vi "Init.vi"(0 "Measurement3D in":refnum<class "Measurement3D.lvclass">, 1 "Instrument 1.lvclass":refnum<class "Instrument.lvclass">, 2 "Instrument 2.lvclass":refnum<class "Instrument.lvclass">, 3 "Instrument 3.lvclass":refnum<class "Instrument.lvclass">, 4 "Inner Loop":T2, 5 "Outer Loop":T1, 7 "error in (no error)":errorcluster) -> (20 "Measurement3D out":refnum<class "Measurement3D.lvclass">, 27 "error out":errorcluster)   [LabVIEW 2014, in "Measurement3D.lvclass"]
uses:
  Measurement3D.lvclass
  Instrument/Instrument/Instrument.lvclass
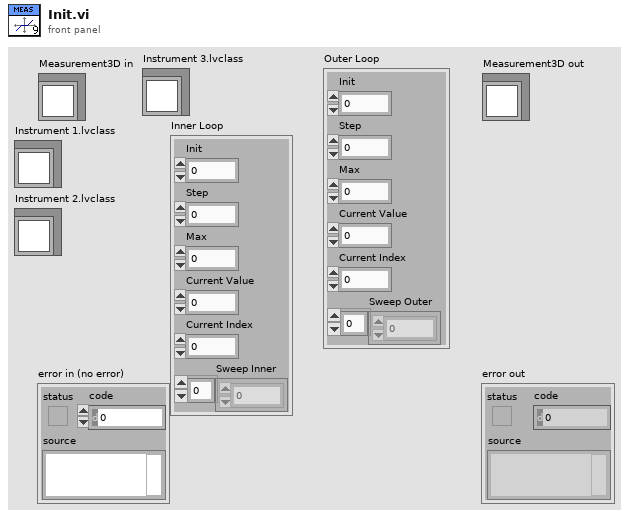
[diagram p1: front panel]
types:
  T1 = cluster{"Init":dbl, "Step":dbl, "Max":dbl, "Current Value":dbl, "Current Index":dbl, "Sweep Outer":dbl[]}
  T2 = cluster{"Init":dbl, "Step":dbl, "Max":dbl, "Current Value":dbl, "Current Index":dbl, "Sweep Inner":dbl[]}
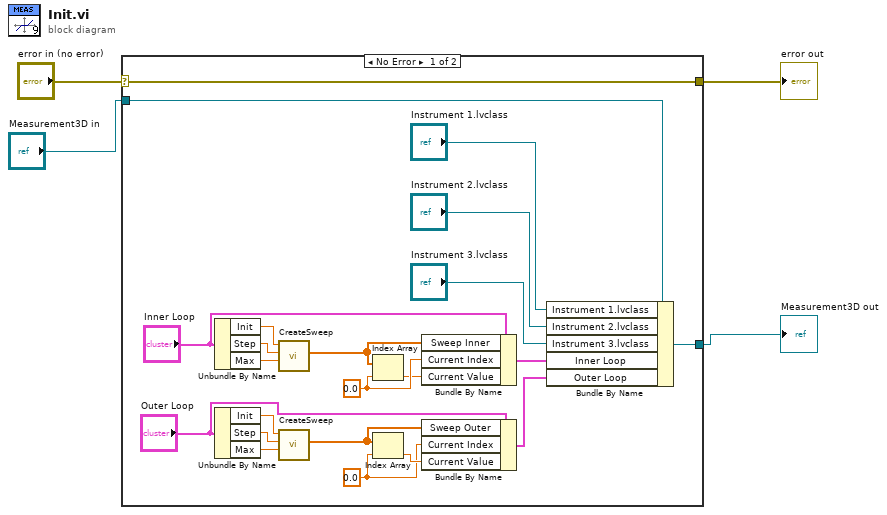
[diagram p0: block diagram]
diagram:
  n1 = case shown="No Error" "error in (no error)" {
    selector: "error in (no error)" -> [w26 w28]
    tunnel: [w26 w28] -> w3
    tunnel: [w21 w27] -> w1
    tunnel: "Measurement3D in" -> [w25 w27]
    frame No Error {
      w6 = 0.0 ("Current Index")
      w9 = 0.0 ("Current Index")
      n2 = Unbundle By Name("Inner Loop") -> ("Init"=w19:dbl, "Step"=w18:dbl, "Max"=w17:dbl)
      n3 = Unbundle By Name("Outer Loop") -> ("Init"=w15:dbl, "Step"=w14:dbl, "Max"=w13:dbl)
      n4 = call "CreateSweep.vi"("Max"=w17, "Step"=w18, "Init Value"=w19) -> ("Array"=w10:dbl[])  [unwired: 8 in]
      n5 = call "CreateSweep.vi"("Max"=w13, "Step"=w14, "Init Value"=w15) -> ("Array"=w5:dbl[])  [unwired: 8 in]
      n6 = Index Array(array=w10, index=w9) -> (element=w8:dbl)
      n7 = Index Array(array=w5, index=w6) -> (element=w7:dbl)
      n8 = Bundle By Name(cluster="Inner Loop", "Sweep Inner"=w10, "Current Index"=w9, "Current Value"=w8) -> (w16:T2)
      n9 = Bundle By Name(cluster="Outer Loop", "Sweep Outer"=w5, "Current Index"=w6, "Current Value"=w7) -> (w11:T1)
      n10 = Bundle By Name(cluster=w25, "Instrument 1.lvclass"="Instrument 1.lvclass", "Instrument 2.lvclass"="Instrument 2.lvclass", "Instrument 3.lvclass"="Instrument 3.lvclass", "Inner Loop"=w16, "Outer Loop"=w11) -> (w21:refnum<class "Measurement3D.lvclass">)
    }
    frame Error {
    }
  }
  "error out" <- w3
  "Measurement3D out" <- w1
